vi "Measure vs B2Dv5beta.vi"() -> ()   [LabVIEW 2009]
doc: "This VI is an example operator panel.\n\nThe VI contains a table for the field values that may be configured manually, or loaded by checking the \"Prompt for File\" box. The data file should contain 3 columns of data, with each column delimited by a tab character.\n\nBefore the VI is executed, set the desired field units and coordinate system. Once the VI is started, follow the directions in the STATUS indicator to operate. Once a field value is achieved, it will be held indefinitely with no user intervention.\n\nThe present field is displayed in the selected units and coordinate system. The present field is queried once per second.\n\nIf a field point is specified that is outside the limits for the magnet, the VI will abort execution."
uses:
  <vilib>/Utility/file.llb/Read From Spreadsheet File (DBL).vi
panel:
  in  "GPIB HP 2":string="13"
  in  "Z-Axis ramp?":bool=TRUE
  in  "Y- Axis ramp?":bool=TRUE
  out "Ist-Länge":dbl=0.009099999999997922
  out "z input":dbl=-3.5494
  out "y input":dbl=-3.5137
  out "Soll-Länge":dbl=4.994429702178218
  in  "FieldRange":dbl=1.0
  in  "Change\nPID\n(DetermineSIMPID.vi)":bool
  in  "X Axis":enum16{"B", "phi"}(ring)=enum."phi"
  in  "Y Axis":T1(ring)=enum."HP (V)"
  out "measured data":dbl[][](array[numeric])
  out "XY Graph":T2(graph)
  in  "Notes:":string="Datum: 5.09.11, Uhrzeit: 17:00, T1.5K, PID LOOP: P 0.5 I 200 D off , PID Dämpfung: P -0.5 D4.4E-5 , Laser 25°, 20mA, AOM 10mA, Sweep 0.09T/min, Winkelsweep 45-225° bei 0.5 T, VectorsM1.txt,  Winkelschritt 2°, mit ManualRamp" caption="Notizen:"
  out "Messfile Refnum":refnum<file>
  in  "Measurement File":path=path "D:/UserData/Matthias/Messungen/STO_LAOR103/110905/110905_R103_0.5T_winkelsweep_M1.txt"
  in  "Sample name:":string="R103"
  in  "HP 1":bool=TRUE
  in  "GPIB HP":string="14"
  in  "HP 2":bool=TRUE
  in  "LI 3":bool
  in  "GPIB L 3":string="8"
  in  "LI 2":bool
  in  "GPIB L 2":string="8"
  in  "LI 1":bool
  in  "GPIB L 1":string="8"
  out "Number of lines":i32=91
  out "Ramp Rate along Vector (T/min)":dbl=0.09 format="%.3f"
  out "Current Ramp Rate Z (T/min)":dbl=0.06396045575747722 format="%.3f"
  out "Current Ramp Rate Y (T/min)":dbl=0.06331713906436233 format="%.3f"
  in  "User defined Ramp Rate (T/min)":bool=TRUE
  in  "User defined Ramp Rate (T/min)":dbl=0.09 format="%.3f"
  in  "Z-Axis Communications Config":T3={"GPIB address"=22, "GPIB bus"=1, "connection ID"=refnum, "IP"="111.111.111.1", "Active Comm Interface"=0, "Serial Port"="", "Programmer Type"=0} {"Programmer Type" items=["Model 430", "Model 420"]; "Active Comm Interface" items=["TCP/IP (Model 430 Only)", "RS232", "IEEE488"]}
  in  "Max Ramp Rate - Y Axis (A/s)":dbl=0.055 format="%.3f"
  in  "Max Ramp Rate - Z Axis (A/s)":dbl=0.19 format="%.3f"
  in  "Magnitude Limit (kG)":dbl=45.1 format="%.3f"
  in  "Y-Axis Communications Config":T3={"GPIB address"=22, "GPIB bus"=1, "connection ID"=refnum, "IP"="111.111.111.2", "Active Comm Interface"=0, "Serial Port"="", "Programmer Type"=0} {"Programmer Type" items=["Model 430", "Model 420"]; "Active Comm Interface" items=["TCP/IP (Model 430 Only)", "RS232", "IEEE488"]}
  out "Cartesian Display (T)":T4={"Y-Axis Field (T)"=-8e-05, "Z-Axis Field (T)"=0.00027} {"Z-Axis Field (T)" format="%.3f"; "Y-Axis Field (T)" format="%.3f"}
  in  "Starting index":i32=92
  in  "Normal color":u32(colorbox)=11711154
  in  "Highlight color":u32(colorbox)=16711680
  in  "Prompt for File?":bool=TRUE
  out "Continue Execution?":bool=TRUE
  out "error out":T5
  in  "error in":T5
  out "STATUS":string="Zeroing vector."
  in  "Ramping Control":u16(ring)=4 items=["NEXT VECTOR", "RAMPING", "HOLDING", "PAUSE", "ZERO"]
  out "Cartesian Display (kG)":T6 {"Z-Axis Field (kG)" format="%.3f"; "Y-Axis Field (kG)" format="%.3f"}
  in  "Field Values":string[][](table)=[["0.5000", "45.0000"], ["0.5000", "47.0000"], ["0.5000", "49.0000"], ["0.5000", "51.0000"], ["0.5000", "53.0000"], ["0.5000", "55.0000"], ["0.5000", "57.0000"], ["0.5000", "59.0000"], ["0.5000", "61.0000"], ["0.5000", "63.0000"], ["0.5000", "65.0000"], ["0.5000", "67.0000"], ["0.5000", "69.0000"], ["0.5000", "71.0000"], ["0.5000", "73.0000"], ["0.5000", "75.0000"], ["0.5000", "77.0000"], ["0.5000", "79.0000"], ["0.5000", "81.0000"], ["0.5000", "83.0000"], ["0.5000", "85.0000"], ["0.5000", "87.0000"], ["0.5000", "89.0000"], ["0.5000", "91.0000"], ["0.5000", "93.0000"], ["0.5000", "95.0000"], ["0.5000", "97.0000"], ["0.5000", "99.0000"], ["0.5000", "101.0000"], ["0.5000", "103.0000"], ["0.5000", "105.0000"], ["0.5000", "107.0000"], ["0.5000", "109.0000"], ["0.5000", "111.0000"], ["0.5000", "113.0000"], ["0.5000", "115.0000"], ["0.5000", "117.0000"], ["0.5000", "119.0000"], ["0.5000", "121.0000"], ["0.5000", "123.0000"], ["0.5000", "125.0000"], ["0.5000", "127.0000"], ["0.5000", "129.0000"], ["0.5000", "131.0000"], ["0.5000", "133.0000"], ["0.5000", "135.0000"], ["0.5000", "137.0000"], ["0.5000", "139.0000"], ["0.5000", "141.0000"], ["0.5000", "143.0000"], ["0.5000", "145.0000"], ["0.5000", "147.0000"], ["0.5000", "149.0000"], ["0.5000", "151.0000"], ["0.5000", "153.0000"], ["0.5000", "155.0000"], ["0.5000", "157.0000"], ["0.5000", "159.0000"], ["0.5000", "161.0000"], ["0.5000", "163.0000"], ["0.5000", "165.0000"], ["0.5000", "167.0000"], ["0.5000", "169.0000"], ["0.5000", "171.0000"], ["0.5000", "173.0000"], ["0.5000", "175.0000"], ["0.5000", "177.0000"], ["0.5000", "179.0000"], ["0.5000", "181.0000"], ["0.5000", "183.0000"], ["0.5000", "185.0000"], ["0.5000", "187.0000"], ["0.5000", "189.0000"], ["0.5000", "191.0000"], ["0.5000", "193.0000"], ["0.5000", "195.0000"], ["0.5000", "197.0000"], ["0.5000", "199.0000"], ["0.5000", "201.0000"], ["0.5000", "203.0000"], ["0.5000", "205.0000"], ["0.5000", "207.0000"], ["0.5000", "209.0000"], ["0.5000", "211.0000"], ["0.5000", "213.0000"], ["0.5000", "215.0000"], ["0.5000", "217.0000"], ["0.5000", "219.0000"], ["0.5000", "221.0000"], ["0.5000", "223.0000"], ["0.5000", "225.0000"]]
  out "Switch Heaters":bool=TRUE
  out "Polar Display (T)":T7 {"Field Magnitude (T)" format="%.3f"; "q (degrees)" format="%.3f"}
  out "Polar Display (kG)":T8 {"Field Magnitude (kG)" format="%.3f"; "q (degrees)" format="%.3f"}
  in  "Coordinate System":u16(ring)=1 items=["Cartesian", "Polar"]
  in  "Magnetic Field Units":u16(ring)=1 items=["kG", "Tesla"]
  # "Vorsicht! Preliminary Measurement Program, watch field limits and pause the power supplies manually when stopping \nthe program!"
  # "Measurement Display"
  # "Measurement Settings"
  # "Magnet Settings"
  # "Max Ramp Rate z: 1.27 T/min\nMax Ramp Rate y: 0.17 T/min"
  # "Devices"
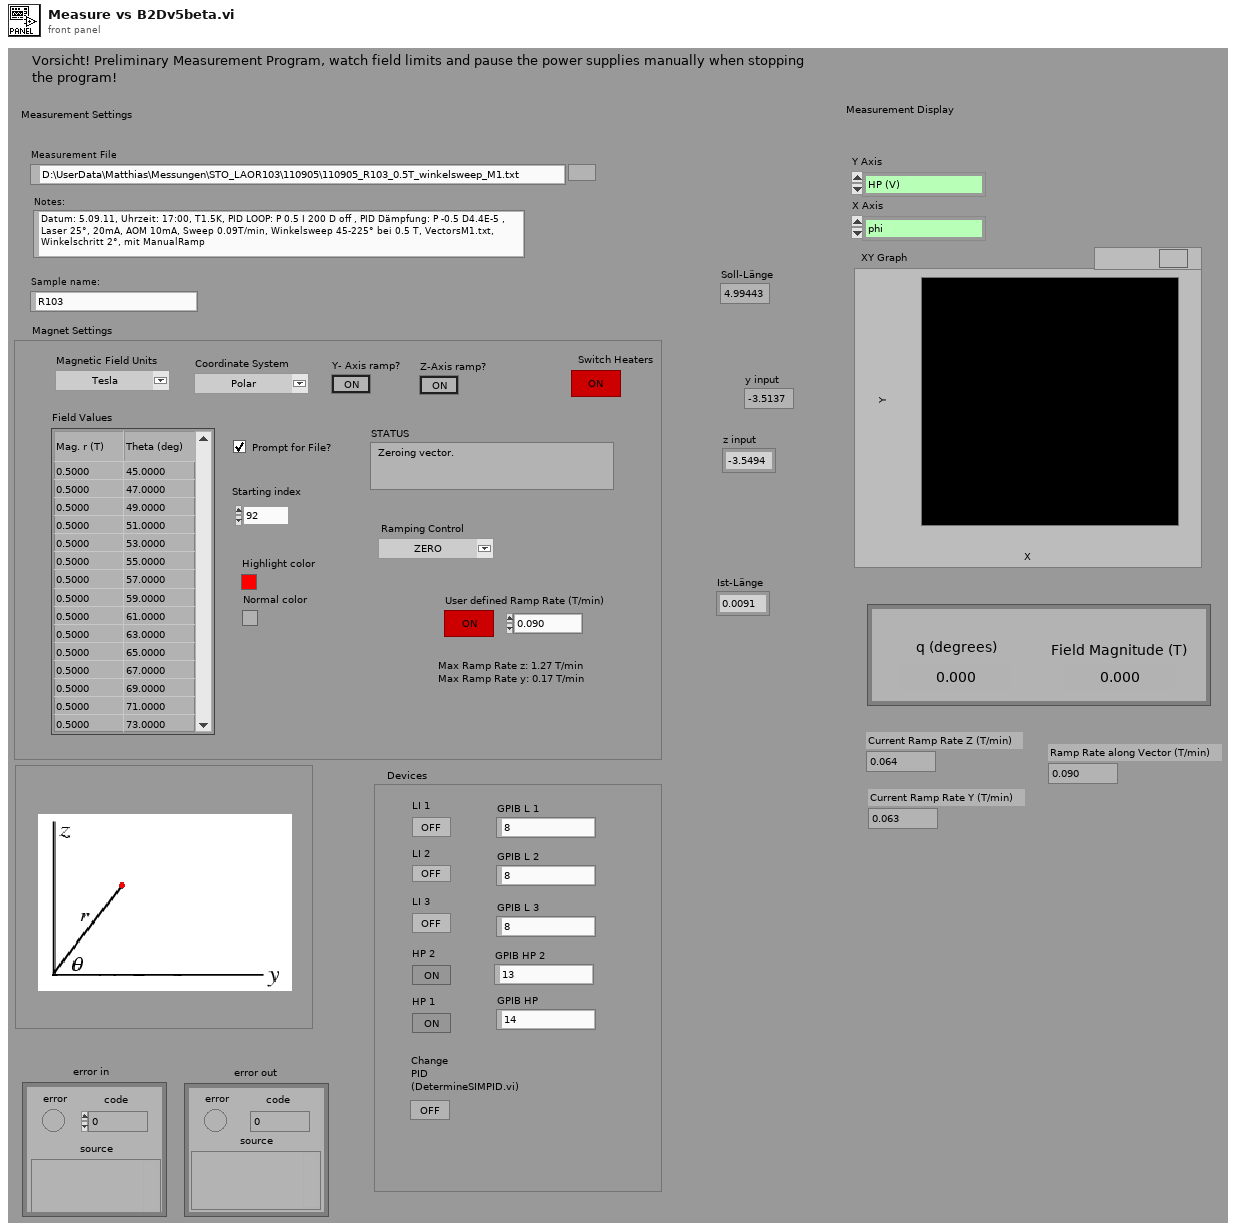
[diagram p1: front panel]
types:
  T1 = enum16{"B", "phi", "LI 1 Vx", "LI 1 phase", "LI 2 Vx", "LI 2 phase", "LI 3 Vx", "LI 3 phase", "LI 4 Vx", "LI 4 phase", "HP (V)"}
  T2 = cluster{"measured data":dbl[], "measured data":dbl[]}
  T3 = cluster{"GPIB address":i16, "GPIB bus":i16, "connection ID":refnum<k5>, "IP":string, "Active Comm Interface":u16, "Serial Port":refnum<visa-resource-name>, "Programmer Type":u16}
  T4 = cluster{"Y-Axis Field (T)":dbl, "Z-Axis Field (T)":dbl}
  T5 = cluster{"error":bool, "code":i32, "source":string}
  T6 = cluster{"Y-Axis Field (kG)":dbl, "Z-Axis Field (kG)":dbl}
  T7 = cluster{"q (degrees)":dbl, "Field Magnitude (T)":dbl}
  T8 = cluster{"q (degrees)":dbl, "Field Magnitude (kG)":dbl}
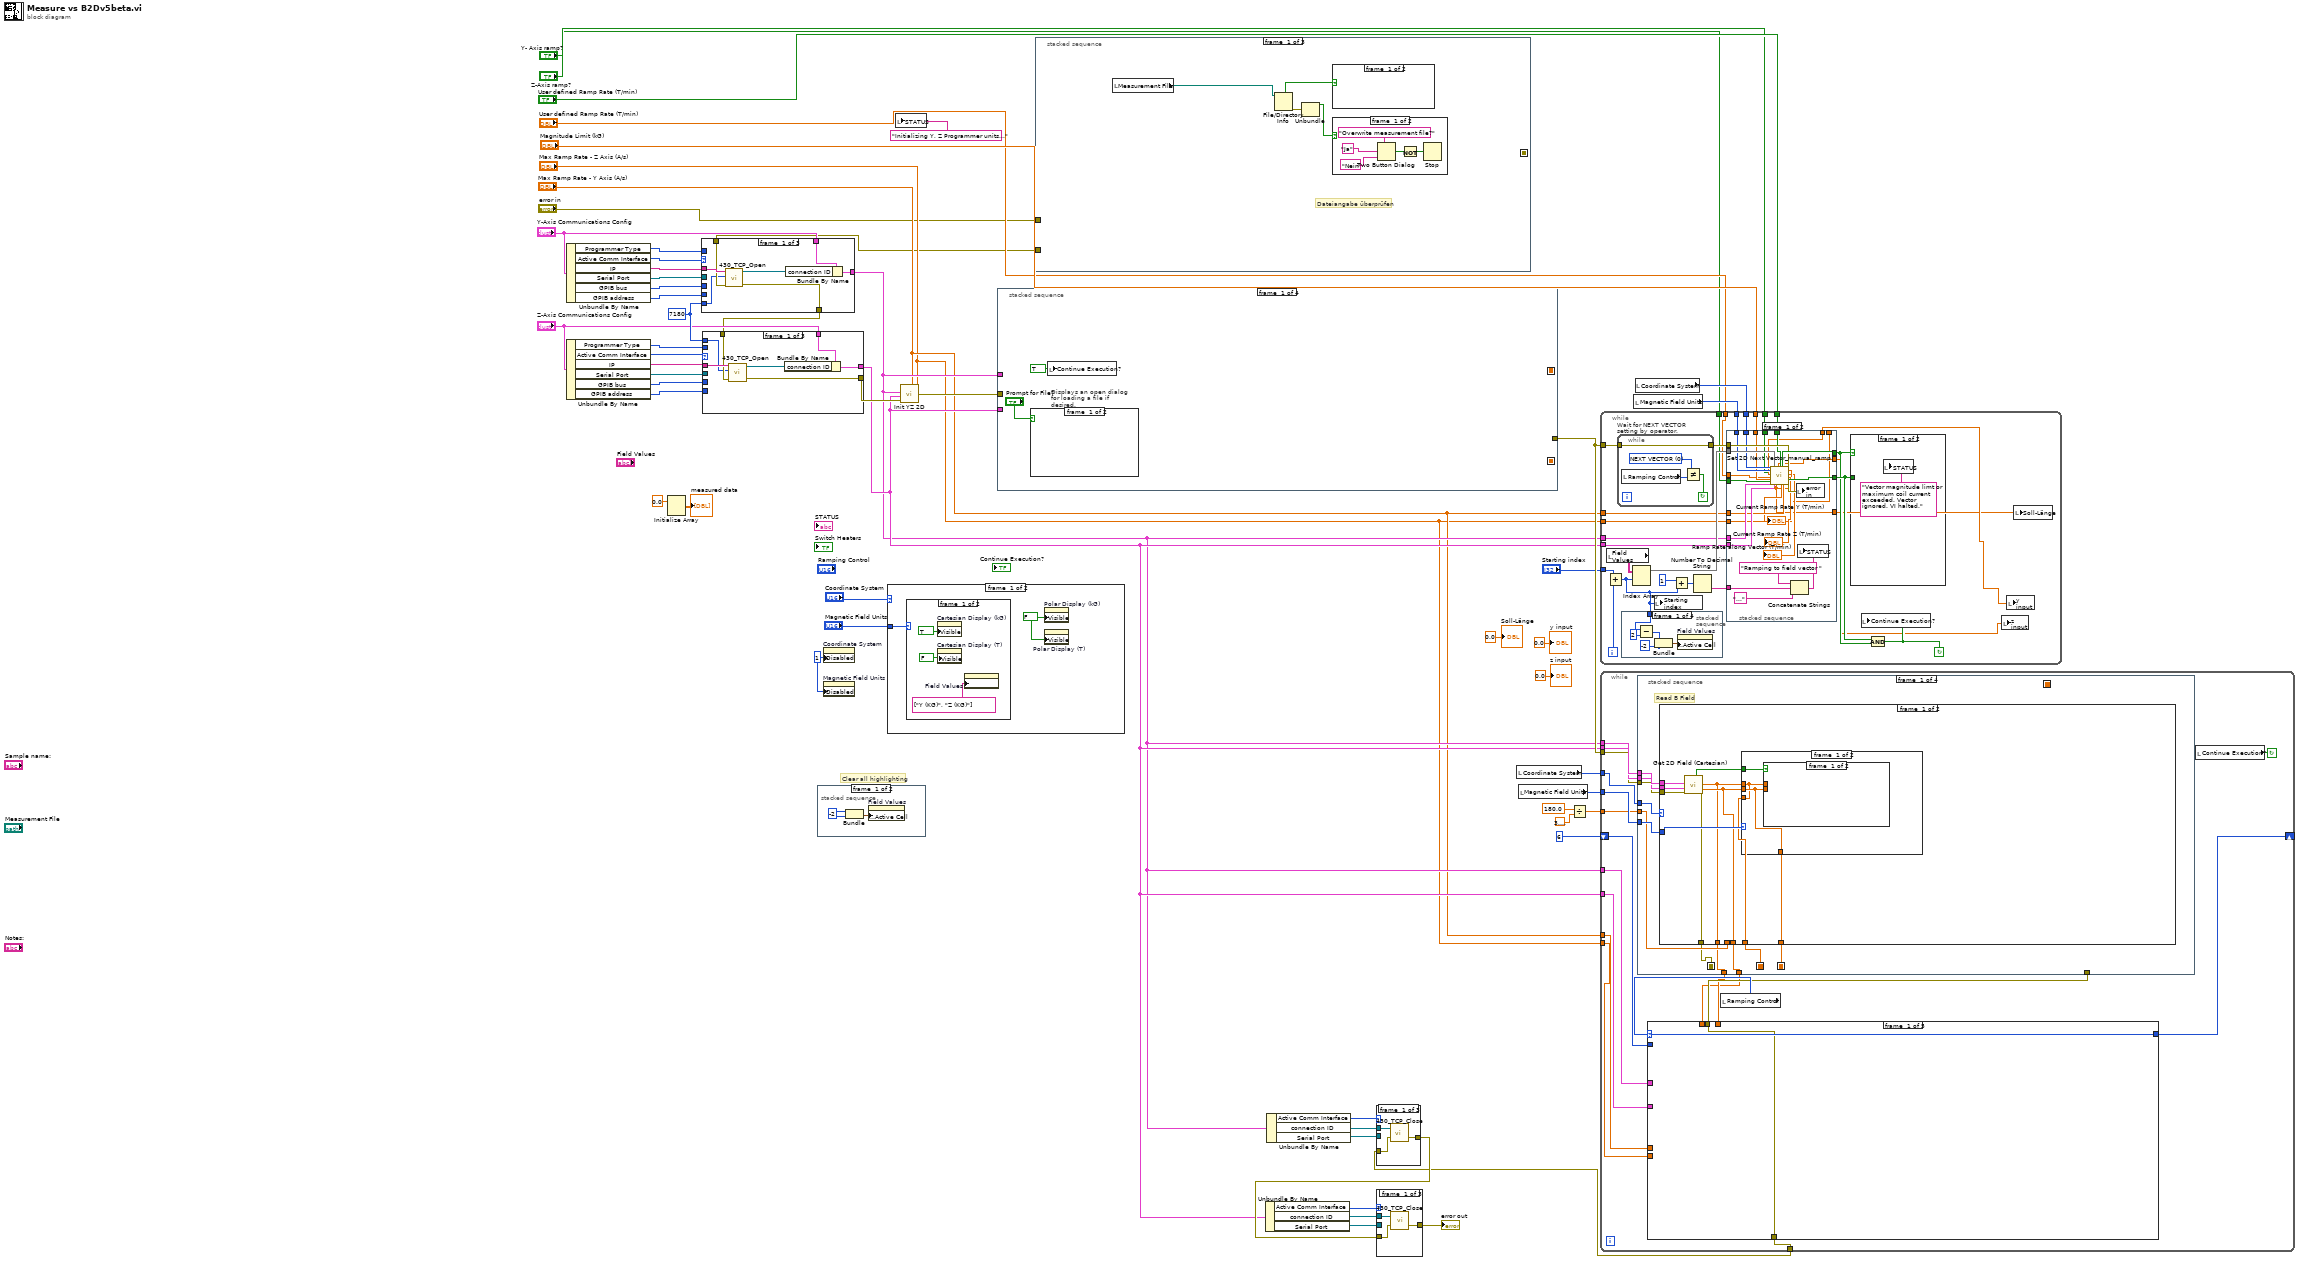
[diagram p0: block diagram]
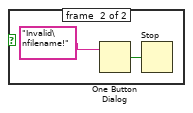
[diagram p3: hidden frame]
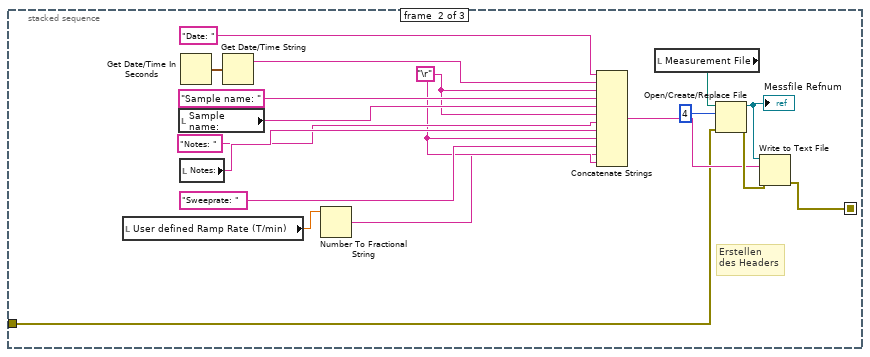
[diagram p4: hidden frame]
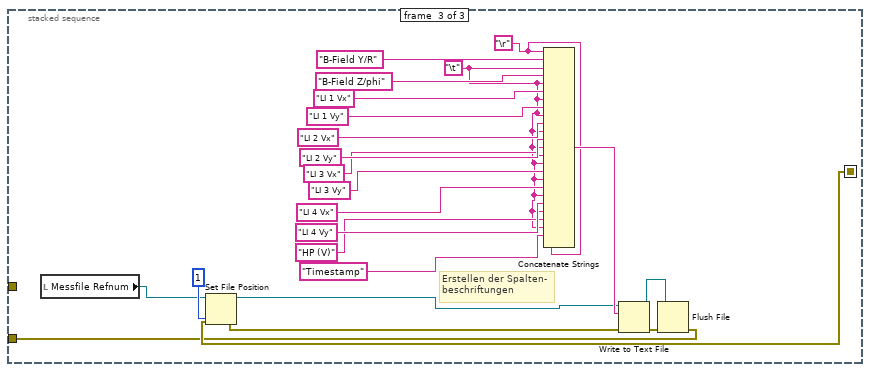
[diagram p5: hidden frame]
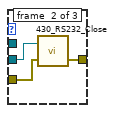
[diagram p6: hidden frame]
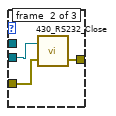
[diagram p8: hidden frame]
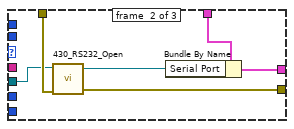
[diagram p10: hidden frame]
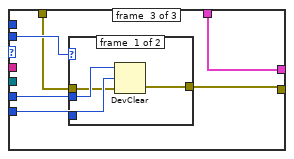
[diagram p11: hidden frame]
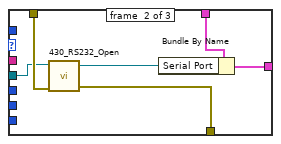
[diagram p13: hidden frame]
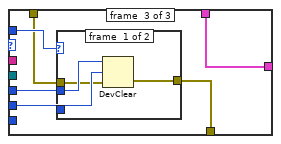
[diagram p14: hidden frame]
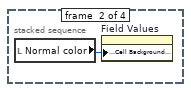
[diagram p16: hidden frame]
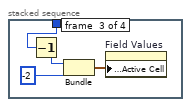
[diagram p17: hidden frame]
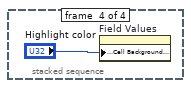
[diagram p18: hidden frame]
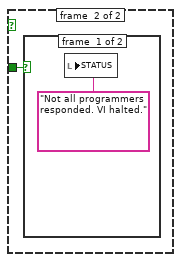
[diagram p19: hidden frame]
diagram:
  w42 = 7180 ("TCP Port")
  w55 = u8 1 ("Write Attribute")
  # "Clear all highlighting"
  n1 = Unbundle By Name("Z-Axis Communications Config") -> ("Programmer Type"=w18:u16, "Active Comm Interface"=w41:u16, "IP"=w38:string, "Serial Port"=w37:refnum<visa-resource-name>, "GPIB bus"=w17:i16, "GPIB address"=w16:i16)
  n2 = Unbundle By Name("Y-Axis Communications Config") -> ("Programmer Type"=w12:u16, "Active Comm Interface"=w40:u16, "IP"=w39:string, "Serial Port"=w36:refnum<visa-resource-name>, "GPIB bus"=w13:i16, "GPIB address"=w14:i16)
  n3 = Initialize Array(0.0 ("element")) -> (→"measured data":dbl[][])  [unwired: 2 in]
  n4 = stacked-sequence {
    frame #0 {
      w58 = -2
      n5 = Bundle(w58, w58) -> (w59:cluster{i32, i32})  [unwired: 1 in]
      n6 = property on="Field Values" class="Tbl (strict)"("Active Cell:Active Cell"=w59) -> ()  [unwired: 2 in, 2 out]
    }
    frame #1 {
      n7 = property on="Field Values" class="Tbl (strict)"("Active Cell:Cell Background Color"="Normal color") -> ()  [unwired: 2 in, 2 out]
    }
  }
  n8 = property on="Coordinate System" class="Ring (strict)"("Disabled"=w55) -> ()  [unwired: 2 in, 2 out]
  n9 = property on="Magnetic Field Units" class="Ring (strict)"("Disabled"=w55) -> ()  [unwired: 2 in, 2 out]
  n10 = case shown="0, Default" "Coordinate System" {
    tunnel: "Magnetic Field Units" -> [w62 w70]
    frame #0 {
      w61 = FALSE ("Write Attribute")
      (unwired) FALSE ("Write Attribute")
      (unwired) TRUE ("Write Attribute")
      n11 = case shown="1" w62 {
        frame #0 {
          n12 = property on="Cartesian Display (kG)" class="Cluster (strict)"("Visible"=TRUE ("Write Attribute")) -> ()  [unwired: 2 in, 2 out]
          n13 = property on="Cartesian Display (T)" class="Cluster (strict)"("Visible"=FALSE ("Write Attribute")) -> ()  [unwired: 2 in, 2 out]
          n14 = property on="Field Values" class="Tbl (strict)"("Column Header Strings[]"=string[] ["Y (KG)", "Z (KG)"] ("Write Attribute")) -> ()  [unwired: 2 in, 2 out]
        }
        frame #1 {
          n15 = property on="Cartesian Display (kG)" class="Cluster (strict)"("Visible"=FALSE ("Write Attribute")) -> ()  [unwired: 2 in, 2 out]
          n16 = property on="Cartesian Display (T)" class="Cluster (strict)"("Visible"=TRUE ("Write Attribute")) -> ()  [unwired: 2 in, 2 out]
          n17 = property on="Field Values" class="Tbl (strict)"("Column Header Strings[]"=string[] ["Y (T)", "Z (T)"] ("Write Attribute")) -> ()  [unwired: 2 in, 2 out]
        }
      }
      n18 = property on="Polar Display (kG)" class="Clust (strict)"("Visible"=w61) -> ()  [unwired: 2 in, 2 out]
      n19 = property on="Polar Display (T)" class="Clust (strict)"("Visible"=w61) -> ()  [unwired: 2 in, 2 out]
    }
    frame #1 {
      (unwired) FALSE ("Write Attribute")
      (unwired) TRUE ("Write Attribute")
      w69 = FALSE ("Write Attribute")
      n20 = case shown="1" w70 {
        frame #0 {
          n21 = property on="Polar Display (kG)" class="Clust (strict)"("Visible"=TRUE ("Write Attribute")) -> ()  [unwired: 2 in, 2 out]
          n22 = property on="Polar Display (T)" class="Clust (strict)"("Visible"=FALSE ("Write Attribute")) -> ()  [unwired: 2 in, 2 out]
          n23 = property on="Field Values" class="Tbl (strict)"("Column Header Strings[]"=string[] ["Mag. r (KG)", "Theta (deg)"] ("Write Attribute")) -> ()  [unwired: 2 in, 2 out]
        }
        frame #1 {
          n24 = property on="Polar Display (kG)" class="Clust (strict)"("Visible"=FALSE ("Write Attribute")) -> ()  [unwired: 2 in, 2 out]
          n25 = property on="Polar Display (T)" class="Clust (strict)"("Visible"=TRUE ("Write Attribute")) -> ()  [unwired: 2 in, 2 out]
          n26 = property on="Field Values" class="Tbl (strict)"("Column Header Strings[]"=string[] ["Mag. r (T)", "Theta (deg)"] ("Write Attribute")) -> ()  [unwired: 2 in, 2 out]
        }
      }
      n27 = property on="Cartesian Display (kG)" class="Cluster (strict)"("Visible"=w69) -> ()  [unwired: 2 in, 2 out]
      n28 = property on="Cartesian Display (T)" class="Cluster (strict)"("Visible"=w69) -> ()  [unwired: 2 in, 2 out]
    }
  }
  n29 = local write "STATUS"("Initializing Y, Z Programmer units..." ("STATUS")) -> ()
  n30 = stacked-sequence {
    seq-local: [_ w88 _] -> [_ _ w107]
    tunnel: "error in" -> [_ w89 _]
    tunnel: [_ _ w106] -> w8
    frame #0 {
      # "Dateiangabe überprüfen"
      n31 = local read "Measurement File"() -> (w80:path)
      n32 = File/Directory Info(path=w80) -> (directory=w78:bool, error out=w79:errorcluster)  [unwired: 1 in, 5 out]
      n33 = Unbundle(w79) -> ("status"=w77:bool)  [unwired: 2 out]
      n34 = case shown="False" w78 {
        frame #0 {
        }
        frame #1 {
          n35 = One Button Dialog(message="Invalid\nfilename!") -> (true=w86:bool)  [unwired: 1 in]
          n36 = Stop(stop? (T)=w86) -> ()
        }
      }
      n37 = case shown="False" w77 {
        frame #0 {
          n38 = Two Button Dialog(message="Overwrite measurement file?", 1:"Nein", 2:"Ja") -> (T button?=w82:bool)
          n39 = Not(x=w82) -> (.not. x?=w81:bool)
          n40 = Stop(stop? (T)=w81) -> ()
        }
        frame #1 {
        }
      }
    }
    frame #1 {
      w92 = "\r"
      # "Erstellen\ndes Headers"
      n41 = local read "User defined Ramp Rate (T/min)"() -> (w91:dbl)
      n42 = local read "Sample name:"() -> (w98:string)
      n43 = local read "Notes:"() -> (w100:string)
      n44 = Get Date/Time In Seconds() -> (seconds since 1Jan1904=w94:timestamp)
      n45 = Get Date/Time String(seconds (now)=w94) -> (date string=w96:string)  [unwired: 2 in, 1 out]
      n46 = Number To Fractional String(number=w91) -> (F-format string=w90:string)  [unwired: 3 in]
      n47 = Concatenate Strings("Date: ", w96, w92, "Sample name: ", w98, w92, "Notes: ", w100, w92, "Sweeprate: ", w90, w92) -> (w104:string)
      n48 = local read "Measurement File"() -> (w101:path)
      n49 = Open/Create/Replace File(file path (use dialog)=w101, error in=w89, operation (0:open)=4) -> (refnum out=w103:refnum<file>, error out=w105:errorcluster)  [unwired: 3 in, 1 out]
      "Messfile Refnum" <- w103
      n50 = Write to Text File(file (use dialog)=w103, text=w104, error in=w105) -> (error out=w88:errorcluster)  [unwired: 1 in, 2 out]
    }
    frame #2 {
      w110 = "\t"
      w108 = "\r"
      # "Erstellen der Spalten-\nbeschriftungen"
      n51 = local read "Messfile Refnum"() -> (w117:refnum<file>)
      n52 = Set File Position(refnum=w117, from (0:start)=1, error in=w107) -> (refnum out=w123:refnum<file>, error out=w125:errorcluster)  [unwired: 1 in]
      n53 = Concatenate Strings(w108, "B-Field Y/R", w110, "B-Field Z/phi", w110, "LI 1 Vx", w110, "LI 1 Vy", w110, "LI 2 Vx", w110, "LI 2 Vy", w110, "LI 3 Vx", w110, "LI 3 Vy", w110, "LI 4 Vx", w110, "LI 4 Vy", w110, "HP (V)", w110, "Timestamp", w108) -> (w124:string)
      n54 = Write to Text File(file (use dialog)=w123, text=w124, error in=w125) -> (refnum out=w127:refnum<file>, error out=w126:errorcluster)  [unwired: 1 in, 1 out]
      n55 = Flush File(refnum=w127, error in=w126) -> (error out=w106:errorcluster)  [unwired: 1 out]
    }
  }
  n56 = case shown="2" w40 {
    tunnel: w39 -> [w135 _ _]
    tunnel: w8 -> [w134 w141 w143]
    tunnel: "Y-Axis Communications Config" -> [w133 w136 w147]
    tunnel: [w131 w139 w147] -> w25
    tunnel: [w130 w140 w142] -> w15
    tunnel: w42 -> [w129 _ _]
    tunnel: w36 -> [_ w137 _]
    tunnel: w14 -> [_ _ w146]
    tunnel: w13 -> [_ _ w145]
    tunnel: w12 -> [_ _ w144]
    frame #0 {
      n57 = call <userlib>:"430_TCP_Open.vi"("IP Address"=w135, "TCP Port"=w129, "error in (no error)"=w134) -> ("connection ID"=w132:refnum<k5>, "error out"=w130:errorcluster)  [unwired: 3 in, 1 out]
      n58 = Bundle By Name(cluster=w133, "connection ID"=w132) -> (w131:T3)
    }
    frame #1 {
      n59 = call <userlib>:"430_RS232_Open.vi"("VISA resource name"=w137, "error in (no error)"=w141) -> ("VISA resource name out"=w138:refnum<visa-resource-name>, "error out"=w140:errorcluster)  [unwired: 5 in]
      n60 = Bundle By Name(cluster=w136, "Serial Port"=w138) -> (w139:T3)
    }
    frame #2 {
      n61 = case shown="0, Default" w144 {
        tunnel: w145 -> [w151 _]
        tunnel: w146 -> [w150 _]
        tunnel: w143 -> [w149 w152]
        tunnel: [w148 w152] -> w142
        frame #0 {
          n62 = DevClear(2:w149, 3:w150, 4:w151) -> (0:w148:errorcluster)  [unwired: 1 out]
        }
        frame #1 {
        }
      }
    }
  }
  n63 = case shown="2" w41 {
    tunnel: w38 -> [w159 _ _]
    tunnel: w15 -> [w158 w165 w167]
    tunnel: [w157 w164 w166] -> w35
    tunnel: "Z-Axis Communications Config" -> [w156 w162 w171]
    tunnel: [w154 w163 w171] -> w26
    tunnel: w42 -> [w153 _ _]
    tunnel: w37 -> [_ w160 _]
    tunnel: w18 -> [_ _ w170]
    tunnel: w17 -> [_ _ w169]
    tunnel: w16 -> [_ _ w168]
    frame #0 {
      n64 = call <userlib>:"430_TCP_Open.vi"("IP Address"=w159, "TCP Port"=w153, "error in (no error)"=w158) -> ("connection ID"=w155:refnum<k5>, "error out"=w157:errorcluster)  [unwired: 3 in, 1 out]
      n65 = Bundle By Name(cluster=w156, "connection ID"=w155) -> (w154:T3)
    }
    frame #1 {
      n66 = call <userlib>:"430_RS232_Open.vi"("VISA resource name"=w160, "error in (no error)"=w165) -> ("VISA resource name out"=w161:refnum<visa-resource-name>, "error out"=w164:errorcluster)  [unwired: 5 in]
      n67 = Bundle By Name(cluster=w162, "Serial Port"=w161) -> (w163:T3)
    }
    frame #2 {
      n68 = case shown="0, Default" w170 {
        tunnel: w169 -> [w175 _]
        tunnel: w168 -> [w174 _]
        tunnel: w167 -> [w173 w176]
        tunnel: [w172 w176] -> w166
        frame #0 {
          n69 = DevClear(2:w173, 3:w174, 4:w175) -> (0:w172:errorcluster)  [unwired: 1 out]
        }
        frame #1 {
        }
      }
    }
  }
  n70 = call <userlib>:"Init YZ 2D.vi"("Max Ramp Rate Z-axis"="Max Ramp Rate - Z Axis (A/s)", "Max Ramp Rate Y-axis"="Max Ramp Rate - Y Axis (A/s)", "error in"=w35, "Z-Axis Communications Config"=w26, "Y-Axis Communications Config"=w25) -> ("error out"=w53:T5)  [unwired: 5 in]
  n71 = stacked-sequence {
    seq-local: [_ w184 _ _] -> [_ _ w231 _]
    seq-local: [_ w183 _ _] -> [_ _ w230 _]
    tunnel: w26 -> [_ w186 _ _]
    tunnel: w53 -> [_ w187 _ _]
    tunnel: [_ w182 _ _] -> w49
    tunnel: w25 -> [_ w185 _ _]
    frame #0 {
      n72 = case "Displays an open dialog for loading a file if desired." shown="True" "Prompt for File?" {
        frame #0 {
        }
        frame #1 {
          n73 = call-poly <vilib>:"Read From Spreadsheet File.vi"() -> ("all rows"=w181:dbl[][])  [unwired: 7 in, 4 out]
          n74 = Number To Fractional String(number=w181, precision (6)=i16 4) -> (F-format string=w180:string[][])  [unwired: 2 in]
          n75 = local write "Field Values"(w180) -> ()
        }
      }
      n76 = local write "Continue Execution?"(TRUE ("Continue Execution?")) -> ()
    }
    frame #1 {
      w195 = u16 3 items=["NEXT VECTOR", "RAMPING", "HOLDING", "PAUSE", "ZERO"] ("Ramping Control")
      n77 = call <userlib>:"Get Switch Present.vi"("error in"=w187, "Communications Config"=w185) -> ("error out"=w191:T5, "Switch Present?"=w192:bool)
      n78 = case shown="True" w192 {
        tunnel: w191 -> [w213 w222]
        tunnel: w185 -> [_ w215]
        tunnel: [0.0 w219] -> w183
        tunnel: [w213 w221] -> w190
        frame #0 {
        }
        frame #1 {
          n79 = call <userlib>:"Get Switch Heater Time.vi"("error in"=w222, "Communications Config"=w215) -> ("error out"=w218:T5, "Switch Heating Time (secs)"=w220:dbl)
          n80 = call <userlib>:"Get Switch Heater.vi"("error in"=w218, "Communications Config"=w215) -> ("error out"=w217:T5, "Switch Heater Indicator"=w216:bool)
          n81 = case shown="False" w216 {
            tunnel: [w227 w228] -> w221
            tunnel: w220 -> [w225 _]
            tunnel: [w225 0.0] -> w219
            tunnel: w217 -> [w223 w228]
            tunnel: w215 -> [w224 _]
            frame #0 {
              n82 = call <userlib>:"Set Switch Heater.vi"("error in"=w223, "Switch Heater Control"=TRUE, "Communications Config"=w224) -> ("error out"=w227:T5)
            }
            frame #1 {
            }
          }
        }
      }
      n83 = call <userlib>:"Get Switch Present.vi"("error in"=w190, "Communications Config"=w186) -> ("error out"=w188:T5, "Switch Present?"=w189:bool)
      n84 = case shown="True" w189 {
        tunnel: w188 -> [w196 w205]
        tunnel: w186 -> [_ w198]
        tunnel: [0.0 w202] -> w184
        tunnel: [w196 w204] -> w182
        frame #0 {
        }
        frame #1 {
          n85 = call <userlib>:"Get Switch Heater Time.vi"("error in"=w205, "Communications Config"=w198) -> ("error out"=w201:T5, "Switch Heating Time (secs)"=w203:dbl)
          n86 = call <userlib>:"Get Switch Heater.vi"("error in"=w201, "Communications Config"=w198) -> ("error out"=w200:T5, "Switch Heater Indicator"=w199:bool)
          n87 = case shown="False" w199 {
            tunnel: [w206 w211] -> w204
            tunnel: w203 -> [w209 _]
            tunnel: [w209 0.0] -> w202
            tunnel: w200 -> [w207 w211]
            tunnel: w198 -> [w208 _]
            frame #0 {
              n88 = call <userlib>:"Set Switch Heater.vi"("error in"=w207, "Switch Heater Control"=TRUE, "Communications Config"=w208) -> ("error out"=w206:T5)
            }
            frame #1 {
            }
          }
        }
      }
      n89 = local write "Ramping Control"(w195) -> ()
      n90 = local write "Switch Heaters"(TRUE ("Switch Heater Control")) -> ()
      n91 = property on="Switch Heaters" class="Boolean (strict)"("Disabled"=u8 1 ("Write Attribute")) -> ()  [unwired: 2 in, 2 out]
    }
    frame #2 {
      n92 = Max & Min(x=w231, y=w230) -> (max(x,y)=w232:dbl)  [unwired: 1 out]
      n93 = local write "STATUS"("Heating switches..." ("STATUS")) -> ()
      n94 = Add(x=w232, y=2) -> (x+y=w236:dbl)
      n95 = property on="Ramping Control" class="Ring (strict)"("Disabled"=u8 1 ("Write Attribute")) -> ()  [unwired: 2 in, 2 out]
      n96 = Multiply(x=w236, y=1000) -> (x*y=w235:dbl)
      n97 = Wait (ms)(milliseconds to wait=w235) -> ()  [unwired: 1 out]
    }
    frame #3 {
      n98 = property on="Ramping Control" class="Ring (strict)"("Disabled"=u8 0 ("Write Attribute")) -> ()  [unwired: 2 in, 2 out]
      n99 = local write "STATUS"("Ready to ramp to first vector. Set Ramping Mode to NEXT VECTOR to begin." ("STATUS")) -> ()
      n100 = local read "Field Values"() -> (w241:string[][])
      n101 = Array Size(array=w241) -> (size(s)=w240:i32[])
      n102 = Index Array(array=w240, index=0) -> (element=→"Number of lines":i32)
    }
  }
  n103 = Unbundle By Name(w26) -> ("Active Comm Interface"=w32:u16, "connection ID"=w31:refnum<k5>, "Serial Port"=w30:refnum<visa-resource-name>)
  n104 = Unbundle By Name(w25) -> ("Active Comm Interface"=w33:u16, "connection ID"=w29:refnum<k5>, "Serial Port"=w28:refnum<visa-resource-name>)
  n105 = local read "Coordinate System"() -> (w50:u16)
  n106 = local read "Magnetic Field Units"() -> (w48:u16)
  n107 = Divide(x=180.0, y=3.141592653589793) -> (x/y=w45:dbl)
  n108 = while {
    shift-left: u16 6 ("Ramping Control") -> [w252]
    shift-right: [w253] -> _
    tunnel: [w255] -> w27
    tunnel: w26 -> [w248]
    tunnel: w25 -> [w249]
    tunnel: w45 -> [w257]
    tunnel: w48 -> [w258]
    tunnel: w49 -> [w259]
    tunnel: w26 -> [w260]
    tunnel: w25 -> [w261]
    tunnel: w50 -> [w262]
    tunnel: "Max Ramp Rate - Y Axis (A/s)" -> [w251]
    tunnel: "Max Ramp Rate - Z Axis (A/s)" -> [w250]
    stop <- w254 continue-if-true
    n109 = stacked-sequence {
      seq-local: [w267 _ _ _] -> [_ _ w373 _]
      seq-local: [w266 _ _ _] -> [_ w342 w370 _]
      seq-local: [w265 _ _ _] -> [_ _ w371 _]
      seq-local: [_ _ w357 _] -> [_ _ _ w436]
      tunnel: w262 -> [w273 _ _ w434]
      tunnel: w261 -> [w272 _ _ _]
      tunnel: w260 -> [w271 _ _ _]
      tunnel: w259 -> [w270 _ _ _]
      tunnel: w258 -> [w269 _ _ _]
      tunnel: w257 -> [w268 _ _ _]
      tunnel: [_ _ w372 _] -> w247
      tunnel: [w264 _ _ _] -> w245
      tunnel: [w263 _ _ _] -> w246
      frame #0 {
        # "Read B Field"
        n110 = case shown="0, Default" w273 {
          tunnel: w272 -> [w283 w308]
          tunnel: w271 -> [w282 w307]
          tunnel: w270 -> [w281 w306]
          tunnel: w269 -> [w280 w305]
          tunnel: w268 -> [_ w304]
          tunnel: [w278 w303] -> w267
          tunnel: [w277 w301] -> w266
          tunnel: [w276 w302] -> w265
          tunnel: [w275 w300] -> w264
          tunnel: [w274 w299] -> w263
          frame #0 {
            n111 = call <userlib>:"Get 2D Field (Cartesian).vi"("Y-Axis Communications Config"=w283, "Z-Axis Communications Config"=w282, "error in"=w281) -> ("All Instruments Responded?"=w279:bool, "Y-Axis Field (kG)"=w274:dbl, "Z-Axis Field (kG)"=w275:dbl, "error out"=w278:T5)  [unwired: 2 in]
            n112 = case shown="0, Default" w280 {
              tunnel: w274 -> [w284 w292]
              tunnel: w275 -> [w285 w293]
              tunnel: w279 -> [w286 w295]
              tunnel: [w285 w291] -> w277
              tunnel: [w284 w290] -> w276
              frame #0 {
                n113 = case shown="True" w286 {
                  tunnel: w284 -> [_ w288]
                  tunnel: w285 -> [_ w287]
                  frame #0 {
                  }
                  frame #1 {
                    n114 = Bundle("Y-Axis Field (kG)"=w288, "Z-Axis Field (kG)"=w287) -> (→"Cartesian Display (kG)":T6)  [unwired: 1 in]
                  }
                }
              }
              frame #1 {
                w294 = 0.1 ("y")
                n115 = Multiply(x=w292, y=w294) -> (x*y=w290:dbl)
                n116 = Multiply(x=w293, y=w294) -> (x*y=w291:dbl)
                n117 = case shown="True" w295 {
                  tunnel: w290 -> [_ w298]
                  tunnel: w291 -> [_ w297]
                  frame #0 {
                  }
                  frame #1 {
                    n118 = Bundle(w298, w297) -> (→"Cartesian Display (T)":cluster{dbl, dbl})  [unwired: 1 in]
                  }
                }
              }
            }
          }
          frame #1 {
            n119 = stacked-sequence {
              tunnel: w308 -> [w323]
              tunnel: w307 -> [w322]
              tunnel: w306 -> [w321]
              tunnel: w305 -> [w320]
              tunnel: w304 -> [w319]
              tunnel: [w317] -> w303
              tunnel: [w316] -> w301
              tunnel: [w315] -> w302
              tunnel: [w310] -> w300
              tunnel: [w309] -> w299
              frame #0 {
                # "Field"
                n120 = call <userlib>:"Get 2D Field (Polar).vi"("Y-Axis Communications Config"=w323, "Z-Axis Communications Config"=w322, "error in"=w321) -> ("All Instruments Responded?"=w318:bool, "Radial (r) Field (kG)"=w313:dbl, "q (radians)"=w314:dbl, "error out"=w317:T5)  [unwired: 2 in]
                n121 = Cosine(x=w314) -> (cos(x)=w311:dbl)
                n122 = Sine(x=w314) -> (sin(x)=w312:dbl)
                n123 = Compound Arithmetic op=MULTIPLY(w313, w312) -> (w310:dbl)
                n124 = case shown="1" w320 {
                  tunnel: w313 -> [w325 w337]
                  tunnel: w314 -> [w327 w336]
                  tunnel: w319 -> [w326 w335]
                  tunnel: w318 -> [w328 w334]
                  tunnel: [w325 w332] -> w316
                  tunnel: [w324 w333] -> w315
                  frame #0 {
                    n125 = Multiply(x=w327, y=w326) -> (x*y=w324:dbl)
                    n126 = case shown="True" w328 {
                      tunnel: w325 -> [_ w329]
                      tunnel: w324 -> [_ w330]
                      frame #0 {
                      }
                      frame #1 {
                        n127 = Bundle(w330, "Radial (r) Field (kG)"=w329) -> (→"Polar Display (kG)":cluster{dbl, "Radial (r) Field (kG)":dbl})  [unwired: 1 in]
                      }
                    }
                  }
                  frame #1 {
                    n128 = Multiply(x=w337, y=0.1) -> (x*y=w333:dbl)
                    n129 = Multiply(x=w336, y=w335) -> (x*y=w332:dbl)
                    n130 = case shown="True" w334 {
                      tunnel: w333 -> [_ w339]
                      tunnel: w332 -> [_ w340]
                      frame #0 {
                      }
                      frame #1 {
                        n131 = Bundle(w340, w339) -> (→"Polar Display (T)":cluster{dbl, dbl})  [unwired: 1 in]
                      }
                    }
                  }
                }
                n132 = Multiply(x=w313, y=w311) -> (x*y=w309:dbl)
              }
            }
          }
        }
      }
      frame #1 {
        # "Change PID"
        n133 = case shown="True" "Change\nPID\n(DetermineSIMPID.vi)" {
          tunnel: w342 -> [_ w347]
          frame #0 {
          }
          frame #1 {
            # "z Field Value"
            n134 = call "CheckFieldRange.vi"("Field Value"=w347) -> ("Field Range"=w344:dbl)  [unwired: 10 in]
            n135 = Equal?(x="FieldRange", y=w344) -> (x = y?=w346:bool)
            n136 = case shown="False" w346 {
              tunnel: w344 -> [w352 w353]
              frame #0 {
                n137 = local write "FieldRange"(w352) -> ()
                n138 = call "DetermineSIMPID.vi"("Field Range"=w352) -> ("D"=w350:string, "P"=w351:string)  [unwired: 7 in, 2 out]
                n139 = call "SIM960ChangeP.vi"("New D Value"=w350, "New P Value"=w351, "Port Num- PID"="1", "GPIB-Adress"="2") -> ()  [unwired: 8 in]
              }
              frame #1 {
                n140 = local write "FieldRange"(w353) -> ()
              }
            }
          }
        }
      }
      frame #2 {
        w356 = u16 2 items=["NEXT VECTOR", "RAMPING", "HOLDING", "PAUSE", "ZERO"] ("Ramping Control")
        # "Zeile in Datei schreiben"
        # "Read and Save Devices"
        n141 = stacked-sequence {
          tunnel: [w385 _ _ _ _ _] -> w369
          tunnel: [w384 _ _ _ _ _] -> w368
          tunnel: [_ w398 _ _ _ _] -> w365
          tunnel: [_ w396 _ _ _ _] -> w364
          tunnel: [_ _ w408 _ _ _] -> w363
          tunnel: [_ _ w407 _ _ _] -> w362
          tunnel: [_ _ _ w418 _ _] -> w361
          tunnel: [_ _ _ w418 _ _] -> w360
          tunnel: [_ _ _ _ w424 _] -> w359
          tunnel: [_ _ _ _ _ w430] -> w358
          frame #0 {
            n142 = case shown="True" "LI 1" {
              tunnel: ["0" ("Antwort2") w392] -> w387
              tunnel: ["0" ("Antwort1") w391] -> w386
              frame #0 {
              }
              frame #1 {
                n143 = call "LI-Ansteuerung.vi"("Frage2"="OUTP? 4", "Frage1"="OUTP? 1", "address string"="GPIB L 1") -> ("Antwort2"=w392:string, "Antwort1"=w391:string)
              }
            }
            n144 = Fract/Exp String To Number(string=w387) -> (number=w384:dbl)  [unwired: 3 in, 1 out]
            n145 = Fract/Exp String To Number(string=w386) -> (number=w385:dbl)  [unwired: 3 in, 1 out]
          }
          frame #1 {
            n146 = case shown="False" "LI 2" {
              tunnel: [w401 w403] -> w397
              tunnel: [w401 w402] -> w399
              frame #0 {
                w401 = "0" ("Antwort1")
              }
              frame #1 {
                n147 = call "LI-Ansteuerung.vi"("Frage2"="OUTP? 4", "Frage1"="OUTP? 1", "address string"="GPIB L 2") -> ("Antwort2"=w403:string, "Antwort1"=w402:string)
              }
            }
            n148 = Fract/Exp String To Number(string=w397) -> (number=w396:dbl)  [unwired: 3 in, 1 out]
            n149 = Fract/Exp String To Number(string=w399) -> (number=w398:dbl)  [unwired: 3 in, 1 out]
          }
          frame #2 {
            n150 = case shown="False" "LI 3" {
              tunnel: [w412 w414] -> w409
              tunnel: [w412 w413] -> w410
              frame #0 {
                w412 = "0" ("Antwort1")
              }
              frame #1 {
                n151 = call "LI-Ansteuerung.vi"("Frage2"="OUTP? 4", "Frage1"="OUTP? 1", "address string"="GPIB L 3") -> ("Antwort2"=w414:string, "Antwort1"=w413:string)
              }
            }
            n152 = Fract/Exp String To Number(string=w410) -> (number=w408:dbl)  [unwired: 3 in, 1 out]
            n153 = Fract/Exp String To Number(string=w409) -> (number=w407:dbl)  [unwired: 3 in, 1 out]
          }
          frame #3 {
            n154 = case shown="False" "HP 2" {
              tunnel: [0.0 ("Voltage") w421] -> w418
              frame #0 {
              }
              frame #1 {
                n155 = call "HP-ReadVoltagev2.vi"("String"="meas:volt:dc? 200,0.001", "HP-Mulitmeter\nGPIB Address"="GPIB HP 2") -> ("Voltage"=w421:dbl)  [unwired: 9 in]
              }
            }
          }
          frame #4 {
            n156 = case shown="True" "HP 1" {
              tunnel: [0.0 ("Voltage") w428] -> w424
              frame #0 {
              }
              frame #1 {
                n157 = call "HP-ReadVoltagev2.vi"("String"="meas:volt:dc? 200,0.001", "HP-Mulitmeter\nGPIB Address"="GPIB HP") -> ("Voltage"=w428:dbl)  [unwired: 9 in]
              }
            }
          }
          frame #5 {
            n158 = Get Date/Time In Seconds() -> (seconds since 1Jan1904=w431:timestamp)
            n159 = To Double Precision Float(number=w431) -> (double precision float=w430:dbl)
          }
        }
        n160 = local read "Ramping Control"() -> (w355:u16)
        n161 = Build Array(w371, w370, w369, w368, w365, w364, w362, w363, w361, w360, w359, w358) -> (w357:dbl[])
        n162 = Array To Spreadsheet String(array=w357, 3:"%f" ("format string")) -> (spreadsheet string=w367:string)  [unwired: 1 in]
        n163 = Equal?(x=w355, y=w356) -> (x = y?=w354:bool)
        n164 = case shown="False" w354 {
          tunnel: w373 -> [w382 w383]
          tunnel: [w381 w383] -> w372
          tunnel: w367 -> [w380 _]
          frame #0 {
            n165 = local read "Messfile Refnum"() -> (w374:refnum<file>)
            n166 = Set File Position(refnum=w374, from (0:start)=1, error in=w382) -> (refnum out=w376:refnum<file>, error out=w377:errorcluster)  [unwired: 1 in]
            n167 = Write to Text File(file (use dialog)=w376, text=w380, error in=w377) -> (refnum out=w379:refnum<file>, error out=w378:errorcluster)  [unwired: 1 in, 1 out]
            n168 = Flush File(refnum=w379, error in=w378) -> (error out=w381:errorcluster)  [unwired: 1 out]
          }
          frame #1 {
          }
        }
      }
      frame #3 {
        n169 = local read "measured data"() -> (w437:dbl[][])
        n170 = Insert Into Array(array=w437, new element=w436) -> (w435:dbl[][])  [unwired: 2 in]
        n171 = case shown="0, Default" w434 {
          tunnel: w435 -> [w453 w467]
          tunnel: "Y Axis" -> [w455 w466]
          tunnel: "X Axis" -> [w443 w465]
          frame #0 {
            n172 = Index Array(array=w453, index (col)=1 ("disabled index (col)")) -> (element=w448:dbl[])  [unwired: 1 in]
            n173 = Index Array(array=w453, index (col)=0 ("disabled index (col)")) -> (element=w447:dbl[])  [unwired: 1 in]
            n174 = Square(x=w448) -> (x^2=w450:dbl[])
            n175 = Square(x=w447) -> (x^2=w451:dbl[])
            n176 = Index Array(array=w453, index (col)=w455) -> (element=w442:dbl[])  [unwired: 1 in]
            n177 = Divide(x=w448, y=w447) -> (x/y=w439:dbl[])
            n178 = Add(x=w451, y=w450) -> (x+y=w449:dbl[])
            n179 = Inverse Tangent(1:w439) -> (0:w438:dbl[])
            n180 = Square Root(x=w449) -> (sqrt(x)=w440:dbl[])
            n181 = Divide(x=w438, y=3.141592653589793) -> (x/y=w445:dbl[])
            n182 = Multiply(x=w445, y=180) -> (x*y=w441:dbl[])
            n183 = case shown="\"B\", Default" w443 {
              tunnel: w442 -> [w458 w461]
              tunnel: w441 -> [_ w460]
              tunnel: w440 -> [w457 _]
              frame #0 {
                n184 = Bundle(w457, "measured data"=w458) -> (w456:cluster{dbl[], "measured data":dbl[]})  [unwired: 1 in]
                n185 = local write "XY Graph"(w456) -> ()
              }
              frame #1 {
                n186 = Bundle(w460, "measured data"=w461) -> (w459:cluster{dbl[], "measured data":dbl[]})  [unwired: 1 in]
                n187 = local write "XY Graph"(w459) -> ()
              }
            }
          }
          frame #1 {
            n188 = Index Array(array=w467, index (col)=w465) -> (element=w464:dbl[])  [unwired: 1 in]
            n189 = Index Array(array=w467, index (col)=w466) -> (element=w463:dbl[])  [unwired: 1 in]
            n190 = Bundle("measured data"=w464, "measured data"=w463) -> (w462:T2)  [unwired: 1 in]
            n191 = local write "XY Graph"(w462) -> ()
          }
        }
        n192 = local write "measured data"(w435) -> ()
      }
    }
    n193 = local read "Ramping Control"() -> (w256:u16)
    n194 = case shown="4" w256 {
      selector: w256 -> [w469 w487 w515 w519 w534]
      tunnel: w249 -> [_ w471 _ w522 w539]
      tunnel: w248 -> [_ w470 _ w521 w538]
      tunnel: [w468 w483 w514 w520 w537] -> w255
      tunnel: [w469 w487 w515 w519 w534] -> w253
      tunnel: w252 -> [_ _ _ w518 w536]
      tunnel: w251 -> [_ _ _ _ w533]
      tunnel: w250 -> [_ _ _ _ w532]
      tunnel: w247 -> [w468 w477 w514 w516 w531]
      tunnel: w246 -> [_ w475 _ _ _]
      tunnel: w245 -> [_ w474 _ _ _]
      frame #0 {
      }
      frame #1 {
        n195 = local read "z input"() -> (w480:dbl)
        n196 = local read "y input"() -> (w481:dbl)
        n197 = local read "Number of lines"() -> (w486:i32)
        n198 = local read "Starting index"() -> (w485:i32)
        n199 = local read "Soll-Länge"() -> (w479:dbl)
        n200 = Less Or Equal?(x=w485, y=w486) -> (x <= y?=w484:bool)
        n201 = call "Calculate_Vector_length_brasse.vi"("Vector 2 z"=w474, "Vector 2 y"=w475, "Vector 1 z"=w480, "Vector 1 y"=w481) -> ("Length"=w482:dbl)  [unwired: 7 in]
        "Ist-Länge" <- w482
        n202 = call "Check 2D Limits_entwurf.vi"("error in"=w477, "Magnitude Limit (kG)"=45.0, "Z-Axis Communications Config"=w470, "Y-Axis Communications Config"=w471, "Z-Axis Field (kG)"=w474, "Y-Axis Field (kG)"=w475) -> ("Within Limits?"=w472:bool, "error out"=w476:T5)  [unwired: 2 in]
        n203 = Greater Or Equal?(x=w482, y=w479) -> (x >= y?=w478:bool)
        n204 = case shown="False" w472 {
          tunnel: w484 -> [_ w500]
          tunnel: [w488 w499] -> w483
          tunnel: w478 -> [_ w498]
          tunnel: w476 -> [w492 w497]
          tunnel: w471 -> [w494 w496]
          tunnel: w470 -> [w490 w495]
          frame #0 {
            w491 = u16 1 items=["RAMP", "PAUSE", "MANUAL UP", "MANUAL DOWN", "ZERO"] ("Ramping Mode")
            w493 = u16 1 items=["RAMP", "PAUSE", "MANUAL UP", "MANUAL DOWN", "ZERO"] ("Ramping Mode")
            # "Beep and pause if outside limits."
            n205 = call "Set Ramping Mode_brasse.vi"("error in"=w492, "Ramping Mode"=w493, "Communications Config"=w494) -> ("error out"=w489:T5)
            n206 = call "Set Ramping Mode_brasse.vi"("error in"=w489, "Ramping Mode"=w491, "Communications Config"=w490) -> ("error out"=w488:T5)
            n207 = call <vilib>:"Beep.vi"() -> ()  [unwired: 12 in]
          }
          frame #1 {
            n208 = case shown="False" w500 {
              tunnel: w497 -> [w504 w511]
              tunnel: [w503 w511] -> w499
              tunnel: w498 -> [_ w510]
              tunnel: w496 -> [w502 _]
              tunnel: w495 -> [w501 _]
              frame #0 {
                w507 = u16 3 items=["NEXT VECTOR", "RAMPING", "HOLDING", "PAUSE", "ZERO"] ("Ramping Control")
                w508 = u16 1 items=["RAMP", "PAUSE", "MANUAL UP", "MANUAL DOWN", "ZERO"] ("Ramping Mode")
                w509 = u16 1 items=["RAMP", "PAUSE", "MANUAL UP", "MANUAL DOWN", "ZERO"] ("Ramping Mode")
                n209 = local write "STATUS"("All Programmers are PAUSED. Set Ramping Mode to NEXT VECTOR to continue." ("STATUS")) -> ()
                n210 = local write "Ramping Control"(w507) -> ()
                n211 = call "Set Ramping Mode_brasse.vi"("error in"=w504, "Ramping Mode"=w508, "Communications Config"=w502) -> ("error out"=w505:T5)
                n212 = call "Set Ramping Mode_brasse.vi"("error in"=w505, "Ramping Mode"=w509, "Communications Config"=w501) -> ("error out"=w503:T5)
              }
              frame #1 {
                n213 = case shown="True" w510 {
                  frame #0 {
                  }
                  frame #1 {
                    n214 = stacked-sequence {
                      frame #0 {
                        w513 = u16 0 items=["NEXT VECTOR", "RAMPING", "HOLDING", "PAUSE", "ZERO"] ("Ramping Control")
                        n215 = local write "Ramping Control"(w513) -> ()
                        n216 = local write "STATUS"("Go to NEXT VECTOR" ("STATUS")) -> ()
                      }
                    }
                  }
                }
              }
            }
          }
        }
      }
      frame #2 {
      }
      frame #3 {
        n217 = Not Equal?(x=w519, y=w518) -> (x != y?=w517:bool)
        n218 = case shown="True" w517 {
          tunnel: w522 -> [_ w530]
          tunnel: w521 -> [_ w529]
          tunnel: [w523 w527] -> w520
          tunnel: w516 -> [w523 w524]
          frame #0 {
          }
          frame #1 {
            w525 = u16 1 items=["RAMP", "PAUSE", "MANUAL UP", "MANUAL DOWN", "ZERO"] ("Ramping Mode")
            # "Beep if outside limits."
            n219 = call <userlib>:"Set Ramping Mode.vi"("error in"=w524, "Ramping Mode"=w525, "Communications Config"=w530) -> ("error out"=w528:T5)
            n220 = call <userlib>:"Set Ramping Mode.vi"("error in"=w528, "Ramping Mode"=w525, "Communications Config"=w529) -> ("error out"=w527:T5)
            n221 = call <vilib>:"Beep.vi"() -> ()  [unwired: 12 in]
            n222 = local write "STATUS"("All Programmers are PAUSED. Set Ramping Mode to NEXT VECTOR to continue." ("STATUS")) -> ()
          }
        }
      }
      frame #4 {
        n223 = Not Equal?(x=w534, y=w536) -> (x != y?=w535:bool)
        n224 = case shown="True" w535 {
          tunnel: w539 -> [_ w548]
          tunnel: w538 -> [_ w547]
          tunnel: [w540 w543] -> w537
          tunnel: w533 -> [_ w546]
          tunnel: w532 -> [_ w545]
          tunnel: w531 -> [w540 w541]
          frame #0 {
          }
          frame #1 {
            w542 = u16 4 items=["RAMP", "PAUSE", "MANUAL UP", "MANUAL DOWN", "ZERO"] ("Ramping Mode")
            n225 = local write "STATUS"("Zeroing vector." ("STATUS")) -> ()
            n226 = call <userlib>:"Set Ramping Mode.vi"("error in"=w541, "Ramping Mode"=w542, "Communications Config"=w548) -> ("error out"=w551:T5)
            n227 = call <userlib>:"Set Ramping Mode.vi"("error in"=w551, "Ramping Mode"=w542, "Communications Config"=w547) -> ("error out"=w544:T5)
            n228 = call <userlib>:"Set Current Ramp Rate.vi"("Communications Config"=w548, "Ramp Rate (A/sec)"=w546, "error in"=w544) -> ("error out"=w549:T5)  [unwired: 2 in]
            n229 = call <userlib>:"Set Current Ramp Rate.vi"("Communications Config"=w547, "Ramp Rate (A/sec)"=w545, "error in"=w549) -> ("error out"=w543:T5)  [unwired: 2 in]
          }
        }
      }
    }
    n230 = local read "Continue Execution?"() -> (w254:bool)
  }
  n231 = case shown="0, Default" w33 {
    tunnel: w29 -> [w554 _ _]
    tunnel: w27 -> [w553 w557 w558]
    tunnel: [w552 w556 w558] -> w34
    tunnel: w28 -> [_ w555 _]
    frame #0 {
      n232 = call <userlib>:"430_TCP_Close.vi"("error in (no error)"=w553, "connection ID"=w554) -> ("error out"=w552:errorcluster)  [unwired: 1 out]
    }
    frame #1 {
      n233 = call <userlib>:"430_RS232_Close.vi"("error in (no error)"=w557, "VISA resource name"=w555) -> ("error out"=w556:errorcluster)  [unwired: 1 in]
    }
    frame #2 {
    }
  }
  n234 = case shown="0, Default" w32 {
    tunnel: w31 -> [w561 _ _]
    tunnel: w34 -> [w560 w564 w565]
    tunnel: [w559 w563 w565] -> w24
    tunnel: w30 -> [_ w562 _]
    frame #0 {
      n235 = call <userlib>:"430_TCP_Close.vi"("error in (no error)"=w560, "connection ID"=w561) -> ("error out"=w559:errorcluster)  [unwired: 1 out]
    }
    frame #1 {
      n236 = call <userlib>:"430_RS232_Close.vi"("error in (no error)"=w564, "VISA resource name"=w562) -> ("error out"=w563:errorcluster)  [unwired: 1 in]
    }
    frame #2 {
    }
  }
  "error out" <- w24
  n237 = local read "Magnetic Field Units"() -> (w51:u16)
  n238 = local read "Coordinate System"() -> (w52:u16)
  n239 = while {
    tunnel: "Starting index" -> [w578]
    tunnel: w26 -> [w584]
    tunnel: w25 -> [w585]
    tunnel: w51 -> [w586]
    tunnel: w52 -> [w587]
    tunnel: w49 -> [w590]
    tunnel: "Max Ramp Rate - Y Axis (A/s)" -> [w574]
    tunnel: "Max Ramp Rate - Z Axis (A/s)" -> [w573]
    tunnel: "Magnitude Limit (kG)" -> [w575]
    tunnel: "User defined Ramp Rate (T/min)" -> [w572]
    tunnel: "User defined Ramp Rate (T/min)" -> [w571]
    tunnel: "Z-Axis ramp?" -> [w567]
    tunnel: "Y- Axis ramp?" -> [w566]
    i -> [w577]
    stop <- w579 continue-if-true
    n240 = local read "Field Values"() -> (w581:string[][])
    n241 = Add(x=w578, y=w577) -> (x+y=w576:i32)
    n242 = while "Wait for NEXT VECTOR setting by operator." {
      tunnel: [w594] -> w589
      tunnel: w590 -> [w594]
      stop <- w595 continue-if-true
      w593 = u16 0 items=["NEXT VECTOR", "RAMPING", "HOLDING", "PAUSE", "ZERO"] ("Ramping Control")
      n243 = local read "Ramping Control"() -> (w596:u16)
      n244 = Not Equal?(x=w593, y=w596) -> (x != y?=w595:bool)
    }
    n245 = stacked-sequence {
      tunnel: w576 -> [w598 _ w604 _]
      frame #0 {
        (unwired) -2
        n246 = Subtract(x=w598, y=2) -> (x-y=w601:i32)
        n247 = Bundle(w601, -2) -> (w599:cluster{i32, i32})  [unwired: 1 in]
        n248 = property on="Field Values" class="Tbl (strict)"("Active Cell:Active Cell"=w599) -> ()  [unwired: 2 in, 2 out]
      }
      frame #1 {
        n249 = local read "Normal color"() -> (w602:u32)
        n250 = property on="Field Values" class="Tbl (strict)"("Active Cell:Cell Background Color"=w602) -> ()  [unwired: 2 in, 2 out]
      }
      frame #2 {
        n251 = Decrement(x=w604) -> (x-1=w603:i32)
        n252 = Bundle(w603, -2) -> (w606:cluster{i32, i32})  [unwired: 1 in]
        n253 = property on="Field Values" class="Tbl (strict)"("Active Cell:Active Cell"=w606) -> ()  [unwired: 2 in, 2 out]
      }
      frame #3 {
        n254 = property on="Field Values" class="Tbl (strict)"("Active Cell:Cell Background Color"="Highlight color") -> ()  [unwired: 2 in, 2 out]
      }
    }
    n255 = Index Array(array=w581, index (row)=w576) -> (element=w588:string[])  [unwired: 1 in]
    n256 = local write "Starting index"(w576) -> ()
    n257 = Add(x=1, y=w576) -> (x+y=w591:i32)
    n258 = Number To Decimal String(number=w591) -> (decimal integer string=w580:string)  [unwired: 1 in]
    n259 = stacked-sequence {
      tunnel: [w636 _] -> w582
      tunnel: [w635 _] -> w583
      tunnel: w589 -> [w631 _]
      tunnel: w588 -> [w630 _]
      tunnel: w587 -> [w629 _]
      tunnel: w586 -> [w628 _]
      tunnel: w585 -> [w627 _]
      tunnel: w584 -> [w626 _]
      tunnel: w580 -> [w625 _]
      tunnel: w575 -> [w623 _]
      tunnel: w574 -> [w622 _]
      tunnel: w573 -> [w617 _]
      tunnel: w572 -> [w621 _]
      tunnel: w571 -> [w620 _]
      tunnel: [w615 _] -> w569
      tunnel: [w614 _] -> w570
      tunnel: [w613 _] -> _
      tunnel: [w613 _] -> w568
      tunnel: w567 -> [w612 _]
      tunnel: w566 -> [w611 _]
      frame #0 {
        n260 = call <userlib>:"Set 2D Next Vector_manual_ramp.vi"("Coordinate System"=w629, "Magnetic Field Units"=w628, "Z-Axis ramp?"=w612, 4:"User defined Ramp Rate (T/min)"=w620, "Magnitude Limit (kG)"=w623, "Y-Axis ramp?"=w611, "Y-Axis Communications Config"=w627, "Input Vector"=w630, "Z-Axis Communications Config"=w626, 14:"User defined Ramp Rate (T/min)"=w621, "Max Ramp Rate - Y Axis (A/s)"=w622, "error in"=w631, "Max Ramp Rate - Z Axis (A/s)"=w617) -> ("Input Vector y (kG)"=w614:dbl, "Soll - Length"=w613:dbl, "Input Vector z (kG)"=w615:dbl, "Y-Axis Ramp Rate (T/min)"=→"Current Ramp Rate Y (T/min)":dbl, "Within Limits?"=w636:bool, "Ramp Rate along Vector (T/min)"=→"Ramp Rate along Vector (T/min)":dbl, "Z-Axis Ramp Rate (T/min)"=→"Current Ramp Rate Z (T/min)":dbl, "All Instruments Responded?"=w635:bool, "error out"=w624:T5)  [unwired: 6 in]
        n261 = Concatenate Strings("Ramping to field vector " ("STATUS"), w625, "..." ("STATUS")) -> (w632:string)
        n262 = local write "error in"(w624) -> ()
        n263 = local write "STATUS"(w632) -> ()
      }
      frame #1 {
        w637 = u16 1 items=["NEXT VECTOR", "RAMPING", "HOLDING", "PAUSE", "ZERO"] ("Ramping Control")
        n264 = local write "Ramping Control"(w637) -> ()
      }
    }
    n265 = case shown="False" w582 {
      tunnel: w583 -> [_ w609]
      frame #0 {
        n266 = local write "STATUS"("Vector magnitude limt or maximum coil current exceeded. Vector ignored. VI halted." ("STATUS")) -> ()
      }
      frame #1 {
        n267 = case shown="False" w609 {
          frame #0 {
            n268 = local write "STATUS"("Not all programmers responded. VI halted." ("STATUS")) -> ()
          }
          frame #1 {
          }
        }
      }
    }
    n269 = Compound Arithmetic op=AND(w583, w582) -> (w579:bool)
    n270 = local write "Continue Execution?"(w579) -> ()
    n271 = local write "z input"(w569) -> ()
    n272 = local write "y input"(w570) -> ()
    n273 = local write "Soll-Länge"(w568) -> ()
  }
  "Soll-Länge" <- 0.0 ("new Vector length")
  "y input" <- 0.0 ("new Vector length")
  "z input" <- 0.0 ("Vector length")
